vi "getMicroscopeParameters.vi"(0 "Microscope in":refnum<class "Microscope.lvclass">, 11 "error in (no error)":errorcluster) -> (4 "Microscope out":refnum<class "Microscope.lvclass">, 6 "Scan Parameters":T4={"x pixels"=256, "x voltage min"=-2.0, "x voltage max"=2.0, "y voltage min"=256.0, "y voltage max"=-2.0, "fill frac"=2.0, "Zoom"=1.0, "BiDi"=FALSE, "scan rate (ms/line)"=2.0} {"Zoom" min=0.0 max=1.0 step=1.0; "fill frac" format="%0.2p"; "y voltage max" format="%0.2p"; "x voltage max" format="%0.2p"; "x voltage min" format="%0.2p"}, 8 "Hardware Settings":T1={"Galvo Channels"="Dev1/ao0:1", "Detector Channels"="Dev1/ai0:2", "Galvo Trigger"="/Dev1/ai/StartTrigger", "Shutter Lines"=["Dev1/port0/line7"], "Max Acquisition Rate"=5000000.0, "Recommended Acquisition Rate"=5000000.0, "Galvo Write Rate"=2500000.0, "Max Timebase Frequency (Hz)"=20000000.0, "MCC Shutter Lines"=[], "Detector Task"="", "Shutter Tasks"=[], "Galvo Task"="", "Digital Image Multiplier"=[100.0, 100.0, -100.0]} {"Max Acquisition Rate" min=0.0 max=5000000.0 step=100000.0}, 10 "Stage Acquire Parameters":T2={"Scan Mode"=enum."Continuous", "Start position mm"=115.0, "End position mm"=112.0, "Velocity um/sec (continuous)"=200.0, "Step size microns (discrete)"=0.0, "Frames to grab (grab)"=200} {"End position mm" format="%_6g"; "Start position mm" format="%_6g"}, 15 "error out":errorcluster)   [LabVIEW 2012, in "Microscope.lvclass"]
doc: "Extracts microscope scan parameters and hardware settings."
uses:
  classes/Microscope.lvclass
  typedefs/Scan Parameters.ctl
  typedefs/Stage Parameters.ctl
  typedefs/ScanMode.ctl
  typedefs/HWsettings.ctl
  classes/Microscope.lvclass/Microscope.ctl
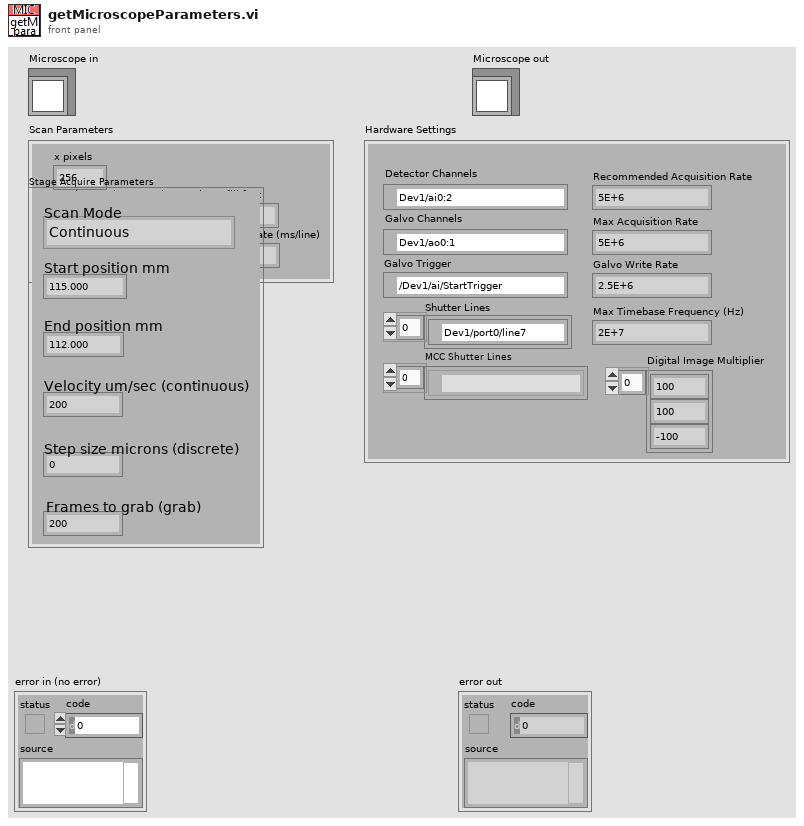
[diagram p1: front panel]
types:
  T1 = typedef "HWsettings.ctl" = cluster{"Galvo Channels":tag, "Detector Channels":tag, "Galvo Trigger":tag, "Shutter Lines":tag[], "Max Acquisition Rate":dbl, "Recommended Acquisition Rate":dbl, "Galvo Write Rate":dbl, "Max Timebase Frequency (Hz)":dbl, "MCC Shutter Lines":refnum<k21>[], "Detector Task":refnum<k21>, "Shutter Tasks":refnum<k21>[], "Galvo Task":refnum<k21>, "Digital Image Multiplier":dbl[]}
  T2 = typedef "Stage Parameters.ctl" = cluster{"Scan Mode":T3, "Start position mm":dbl, "End position mm":dbl, "Velocity um/sec (continuous)":dbl, "Step size microns (discrete)":dbl, "Frames to grab (grab)":i32}
  T3 = typedef "ScanMode.ctl" = enum16{"None", "Continuous", "Point Scan (CH3 cursor)", "Point Scan Move (CH3 cursor)", "Grab", "Grab Move Stage", "Grab Move Z-stage", "Cont. Move Z-stage", "Spec Move Stage", "Spec Move Cont", "Surf Calib"}
  T4 = typedef "Scan Parameters.ctl" = cluster{"x pixels":i32, "x voltage min":dbl, "x voltage max":dbl, "y voltage min":dbl, "y voltage max":dbl, "fill frac":dbl, "Zoom":dbl, "BiDi":bool, "scan rate (ms/line)":dbl}
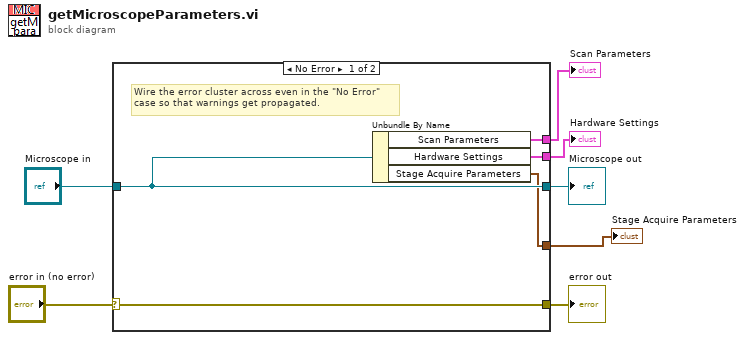
[diagram p0: block diagram]
diagram:
  n1 = case shown="No Error" "error in (no error)" {
    selector: "error in (no error)" -> [w12 w14]
    tunnel: [w12 w14] -> w6
    tunnel: [w11 w13] -> w4
    tunnel: "Microscope in" -> [w11 w13]
    tunnel: [w10 _] -> w3
    tunnel: [w9 _] -> w1
    tunnel: [w8 _] -> w2
    frame No Error {
      # "Wire the error cluster across even in the \"No Error\"\ncase so that warnings get propagated."
      n2 = Unbundle By Name(w11) -> ("Scan Parameters"=w10:T4, "Hardware Settings"=w9:T1, "Stage Acquire Parameters"=w8:T2)
    }
    frame Error {
    }
  }
  "error out" <- w6
  "Microscope out" <- w4
  "Scan Parameters" <- w3
  "Stage Acquire Parameters" <- w2
  "Hardware Settings" <- w1
